vi "labview TX Code.vi"() -> ()   [LabVIEW 2014]
uses:
  <vilib>/Instr/_visa.llb/VISA Configure Serial Port (Instr).vi
  <userlib>/_OpenG.lib/labpython/labpython.llb/PYTHON Set Integer Data__ogtk.vi
  <userlib>/_OpenG.lib/labpython/labpython.llb/PYTHON Set Float Data__ogtk.vi
  <userlib>/_OpenG.lib/labpython/labpython.llb/PYTHON Get Integer Data__ogtk.vi
panel:
  in  "key":dbl
  out "error out 2":errorcluster
  in  "decrypt Python script":string
  in  "error in (no error) 2":errorcluster
  in  "VISA resource name":refnum<visa-resource-name>
  in  "error in (no error)":errorcluster
  out "error out":errorcluster
  in  "stop":bool
  out "binarycode":string
  in  "request":bool
  in  "timeout (100 ms)":u32=10000
  in  "baud rate (115200)":u32=9600
  in  "data bits (8)":u16=8 min=5 max=8 step=1
  in  "parity (0:none)":enum16{"None", "Odd", "Even", "Mark", "Space"}(ring)
  in  "flow control (0:none)":u16(ring) items=["None", "XON/XOFF", "RTS/CTS", "XON/XOFF & RTS/CTS", "DTR/DSR", "XON/XOFF & DTR/DSR"]
  in  "stop bits (10: 1 bit)":u16(ring)=10 items=["1.0"=10, "1.5"=15, "2.0"=20]
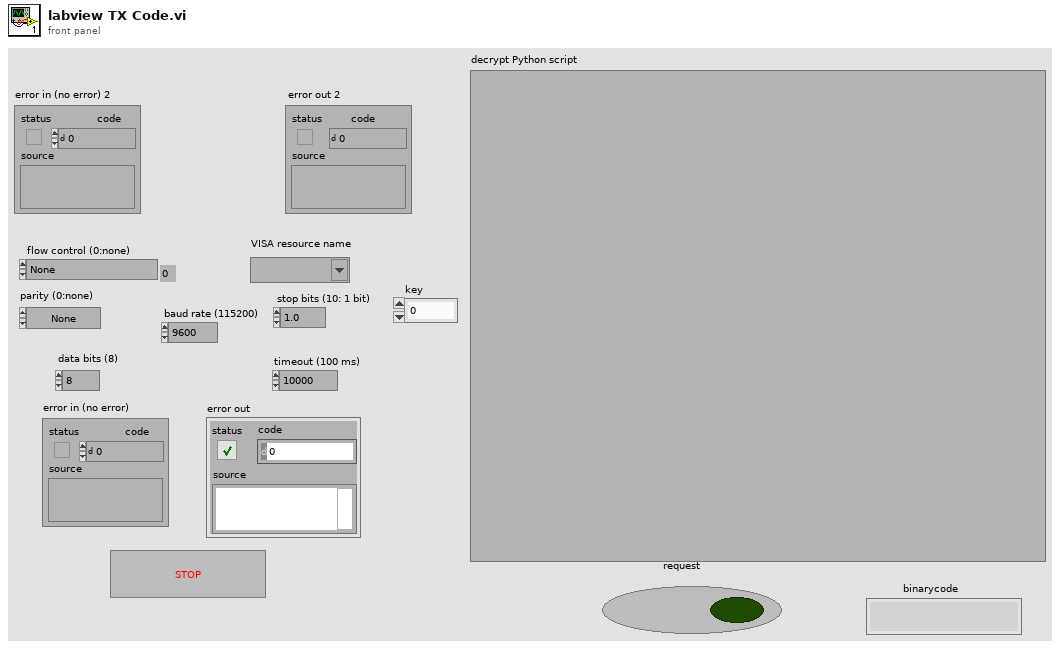
[diagram p1: front panel]
types:
  T1 = typedef "PYTHON Session Refnum__ogtk.ctl" = refnum<k1>
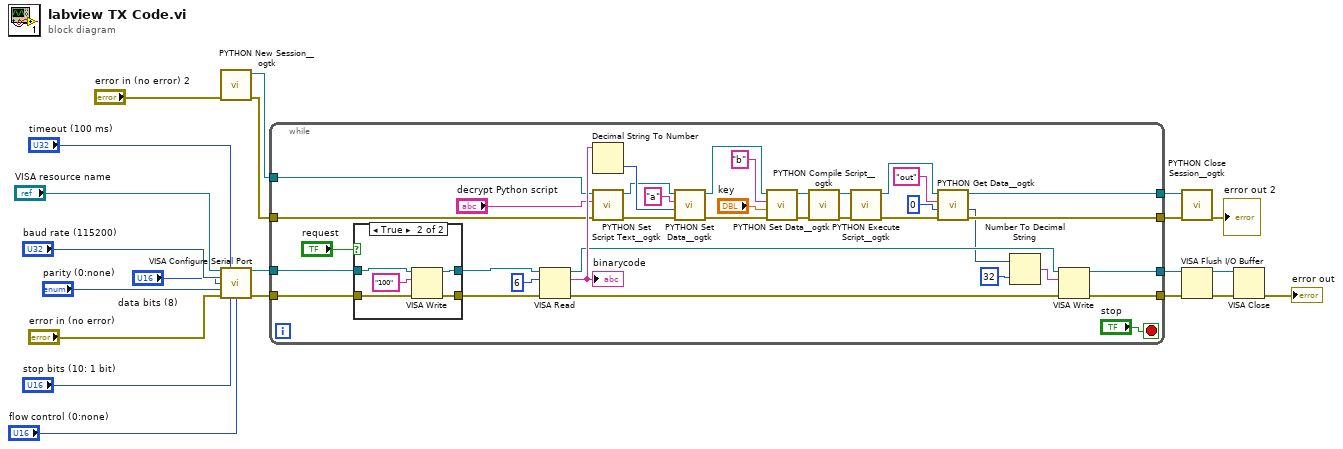
[diagram p0: block diagram]
diagram:
  n1 = call <userlib>:"PYTHON New Session__ogtk.vi"("error in (no error)"="error in (no error) 2") -> ("error out"=w4:errorcluster, "Python Session"=w5:T1)  [unwired: 5 in]
  n2 = call-poly "VISA Configure Serial Port"("VISA resource name"="VISA resource name", "timeout (10sec)"="timeout (100 ms)", "baud rate (9600)"="baud rate (115200)", "data bits (8)"="data bits (8)", "parity (0:none)"="parity (0:none)", "error in (no error)"="error in (no error)", "stop bits (10: 1 bit)"="stop bits (10: 1 bit)", "flow control (0:none)"="flow control (0:none)") -> ("VISA resource name out"=w13:refnum<visa-resource-name>, "error out"=w14:errorcluster)  [unwired: 6 in]
  n3 = while {
    tunnel: w13 -> [w52]
    tunnel: w14 -> [w53]
    tunnel: [w31] -> w20
    tunnel: [w33] -> w18
    tunnel: w5 -> [w41]
    tunnel: w4 -> [w49]
    tunnel: [w43] -> w3
    tunnel: [w42] -> w2
    stop <- "stop" stop-if-true
    n4 = case shown="True" "request" {
      tunnel: w53 -> [w59 w64]
      tunnel: [w59 w63] -> w50
      tunnel: [w58 w62] -> w51
      tunnel: w52 -> [w58 w60]
      frame False {
      }
      frame True {
        n5 = VISA Write(VISA resource name=w60, write buffer="100", error in (no error)=w64) -> (VISA resource name out=w62:refnum<visa-resource-name>, error out=w63:errorcluster)  [unwired: 1 out]
      }
    }
    n6 = VISA Read(VISA resource name=w51, byte count=6, error in (no error)=w50) -> (VISA resource name out=w34:refnum<visa-resource-name>, read buffer=w55:string, error out=w32:errorcluster)  [unwired: 1 out]
    "binarycode" <- w55
    n7 = Decimal String To Number(string=w55) -> (number=w39:i32)  [unwired: 2 in, 1 out]
    n8 = call <userlib>:"PYTHON Set Script Text__ogtk.vi"("error in (no error)"=w49, "script text"="decrypt Python script", "Python Session in"=w41) -> ("error out"=w48:errorcluster, "Python Session out"=w37:T1)  [unwired: 3 in]
    n9 = call-poly <userlib>:"PYTHON Set Data__ogtk.vi"("error in (no error)"=w48, "value"=w39, "variable name"="a", "Python Session in"=w37) -> ("error out"=w29:errorcluster, "Python Session out"=w30:T1)  [unwired: 2 in]
    n10 = call-poly <userlib>:"PYTHON Set Data__ogtk.vi"("error in (no error)"=w29, "value"="key", "variable name"="b", "Python Session in"=w30) -> ("error out"=w27:errorcluster, "Python Session out"=w28:T1)  [unwired: 2 in]
    n11 = call <userlib>:"PYTHON Compile Script__ogtk.vi"("error in (no error)"=w27, "Python Session in"=w28) -> ("error out"=w35:errorcluster, "Python Session out"=w36:T1)  [unwired: 4 in]
    n12 = call <userlib>:"PYTHON Execute Script__ogtk.vi"("error in (no error)"=w35, "Python Session in"=w36) -> ("error out"=w46:errorcluster, "Python Session out"=w47:T1)  [unwired: 4 in]
    n13 = call-poly <userlib>:"PYTHON Get Data__ogtk.vi"("error in (no error)"=w46, "data type"=0, "variable name"="out", "Python Session in"=w47) -> ("error out"=w42:errorcluster, "value"=w24:i32, "Python Session out"=w43:T1)  [unwired: 1 in]
    n14 = Number To Decimal String(number=w24, width (-)=i16 32) -> (decimal integer string=w23:string)
    n15 = VISA Write(VISA resource name=w34, write buffer=w23, error in (no error)=w32) -> (VISA resource name out=w33:refnum<visa-resource-name>, error out=w31:errorcluster)  [unwired: 1 out]
  }
  n16 = call <userlib>:"PYTHON Close Session__ogtk.vi"("error in (no error)"=w2, "Python Session in"=w3) -> ("error out"=→"error out 2":errorcluster)  [unwired: 5 in]
  n17 = VISA Flush I/O Buffer(VISA resource name=w18, error in (no error)=w20) -> (VISA resource name out=w19:refnum<visa-resource-name>, error out=w21:errorcluster)  [unwired: 1 in]
  n18 = VISA Close(VISA resource name=w19, error in (no error)=w21) -> (error out=→"error out":errorcluster)
